vi "Real_Time_Main_Final.vi"() -> ()   [LabVIEW 2024]
uses:
  <instrlib>/niScope/Controls/niScope trigger source.ctl
  <vilib>/Platform/TimedLoop/XDataNode/timing_clust.ctl
  <vilib>/Platform/TimedLoop/XDataNode/nitl_modes.ctl
  <vilib>/Platform/TimedLoop/XDataNode/wakeup.ctl
  <instrlib>/niScope/Controls/niScope vertical coupling.ctl
  <instrlib>/niScope/Controls/niScope timestamp type.ctl
  <instrlib>/niScope/Configure/Trigger/niScope Configure Trigger Edge.vi
  <instrlib>/niScope/Acquire/Fetch/niScope Fetch WDT.vi
  <vilib>/platform/TimedLoop/XDataNode/XDataNode.xnode
  <vilib>/Platform/TimedLoop/XDataNode/XDNodeRunTimeDep.lvlib
panel:
  in  "stop 2":bool
  in  "Fetch:Fetch Relative To":i32(ring)=482 items=["Start"=482, "Trigger"=483, "Pretrigger"=477, "Now"=481, "Read Pointer"=388]
  in  "stop":bool
  out "error out":errorcluster
  out "Horizontal:Actual Sample Rate":dbl
  in  "channels":string="0"
  out "# of Points Fetched":i32
  out "# of Chunks Fetched":i32
  in  "trigger source":T1="0" caption="trigger source (Channel 0)"
  in  "Resource Name":refnum<k15>="Dev1" caption="Resource Name(s)"
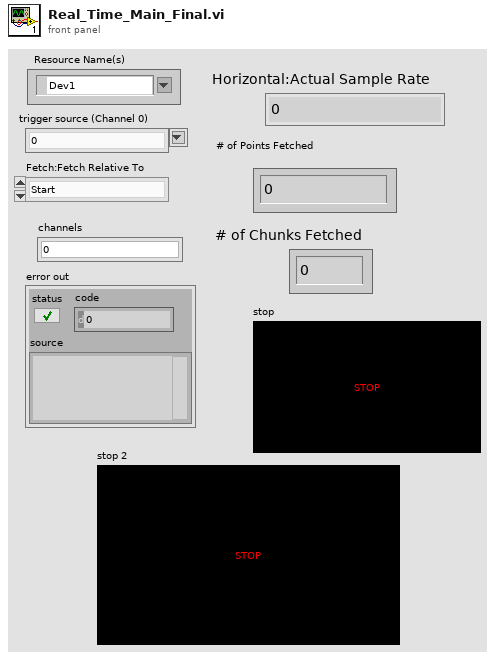
[diagram p1: front panel]
types:
  T1 = typedef "niScope trigger source.ctl" = string
  T2 = typedef "XDNodeRunTimeDep.lvlib/timing_clust.ctl" = cluster{"Expected End [f-1]":u64, "Actual End [f-1]":u64, "Finished Late? [f-1]":bool, "Expected End [i-1]":u64, "Actual End [i-1]":u64, "Finished Late? [i-1]":bool, "Expected Start [i]":u64, "Actual Start [i]":u64, "Expected Start [f]":u64, "Actual Start [f]":u64, "Source Name":string, "Structure Name":string, "Period":i64, "Deadline":i64, "Offset":i64, "Start":i64, "Priority":i32, "Timeout":i32, "Mode":T3, "Wakeup Reason":T4, "Error":errorcluster, "Source Type":string, "Secondary Source Type":string, "Global End Time":u64, "Global Start Time":u64, "Frame Duration":u64, "Iteration Duration":u64, "Assigned CPU":i32, "I/O Scan Engine Mode":u32}
  T3 = typedef "XDNodeRunTimeDep.lvlib/nitl_modes.ctl" = enum32{"No Change", "Process missed periods, maintain original phase", "Discard missed periods, maintain original phase", "Process missed periods, ignore original phase", "Discard missed periods, ignore original phase"}
  T4 = typedef "XDNodeRunTimeDep.lvlib/wakeup.ctl" = enum32{"Normal", "Aborted", "Asynchronous wakeup", "Timing source error", "Timed loop error", "Timeout"}
  T5 = typedef "niScope timestamp type.ctl" = i32
  T6 = typedef "niScope vertical coupling.ctl" = i32
  T7 = cluster{"actualSamples":i32, "absoluteInitialX":dbl, "relativeInitialX":dbl, "xIncrement":dbl, "offset":dbl, "gain":dbl, "reserved1":dbl, "reserved2":dbl}
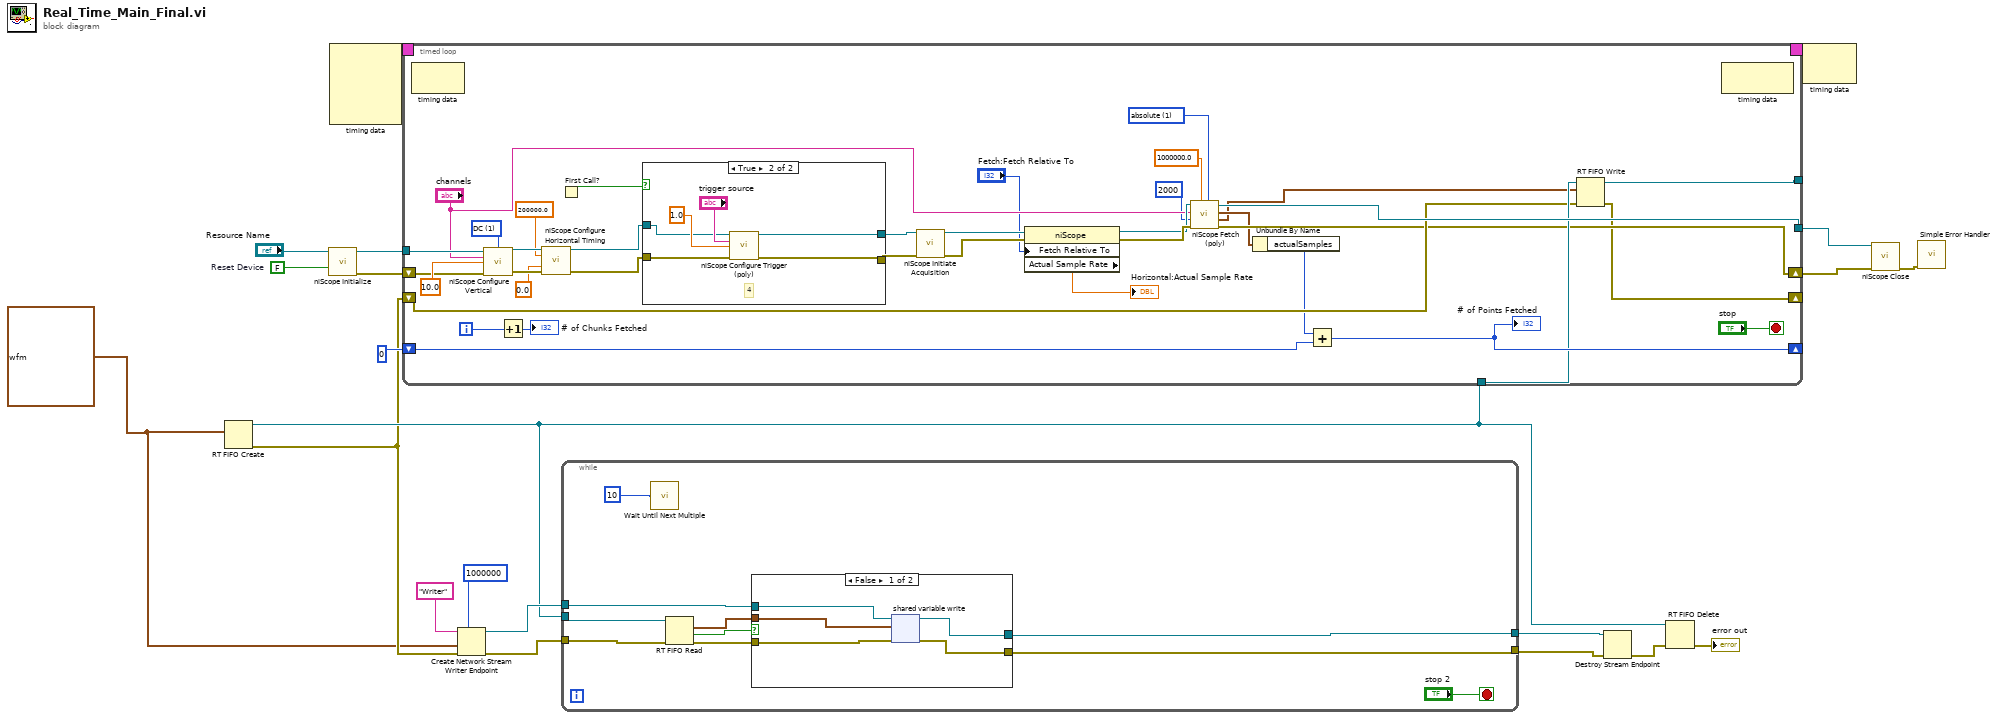
[diagram p0: block diagram]
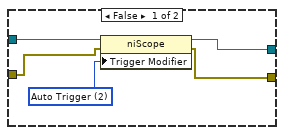
[diagram p3: hidden frame]
diagram:
  w1 = waveform(dbl) {"t0"=timestamp(0 s since 1904-01-01), "dt"=1.0, "Y"=[]}
  w21 = FALSE  # Reset Device
  n1 = RT FIFO Create(1:w1) -> (8:w6:refnum<k33>, 11:w3:errorcluster)  [unwired: 7 in, 1 out]
  n2 = call <instrlib>:"niScope Initialize.vi"("resource name"="Resource Name", "reset device"=w21) -> ("instrument handle"=w15:refnum<k15>, "error out"=w5:errorcluster)  [unwired: 12 in]
  n3 = node-c288() -> (w19:T2)  [unwired: 4 in]
  n4 = timed-loop {
    timing: w19 -> [_]
    timing-out: [_] -> w18
    tunnel: [w49] -> w17
    shift-right: [w47] -> _
    shift-left: 0 -> [w48]
    tunnel: w15 -> [w38]
    tunnel: w6 -> [w34]
    tunnel: [w33] -> _
    shift-right: [w26] -> _
    shift-left: w3 -> [w29]
    shift-right: [w27] -> w4
    shift-left: w5 -> [w28]
    i -> [w46]
    stop <- "stop" stop-if-true
    w23 = T5 1 items=["relative", "absolute"] ("timestamp Type")
    w42 = T6 1 items=["AC", "DC", "Ground"] ("vertical coupling")
    n5 = node-c288() -> ()  [unwired: 1 in, 1 out]
    n6 = call <instrlib>:"niScope Configure Vertical.vi"("instrument handle"=w38, "vertical coupling"=w42, "channels"="channels", "vertical range"=10.0, "error in"=w28) -> ("instrument handle out"=w45:refnum<k15>, "error out"=w39:errorcluster)  [unwired: 9 in]
    n7 = Increment(x=w46) -> (x+1=→"# of Chunks Fetched":i32)
    n8 = call <instrlib>:"niScope Configure Horizontal Timing.vi"("instrument handle"=w45, "min sample rate"=200000.0, "reference position"=0.0, "error in"=w39) -> ("instrument handle out"=w40:refnum<k15>, "error out"=w41:errorcluster)  [unwired: 10 in]
    n9 = First Call?() -> (First Call?: T/F=w57:bool)
    n10 = case shown="True" w57 {
      tunnel: [w62 w67] -> w58
      tunnel: [w63 w66] -> w51
      tunnel: w41 -> [w60 w65]
      tunnel: w40 -> [w59 w64]
      frame False {
        w61 = 2 items=["None"=1, "Auto Trigger"=2] ("Triggering:Trigger Modifier")
        n11 = property class="niScope"(reference=w59, error in=w60, "Trigger Modifier"=w61) -> (reference out=w63:refnum<k15>, error out=w62:errorcluster)
      }
      frame True {
        # "4"
        n12 = call-poly <instrlib>:"niScope Configure Trigger (poly).vi"("instrument handle"=w64, "trigger source"="trigger source", "trigger level"=1.0, "error in"=w65) -> ("instrument handle out"=w66:refnum<k15>, "error out"=w67:errorcluster)  [unwired: 10 in]
      }
    }
    n13 = call <instrlib>:"niScope Initiate Acquisition.vi"("instrument handle"=w51, "error in"=w58) -> ("instrument handle out"=w52:refnum<k15>, "error out"=w56:errorcluster)  [unwired: 12 in]
    n14 = property class="niScope"(reference=w52, error in=w56, "Fetch Relative To"="Fetch:Fetch Relative To") -> (reference out=w53:refnum<k15>, error out=w54:errorcluster, "Actual Sample Rate"=→"Horizontal:Actual Sample Rate":dbl)
    n15 = call-poly <instrlib>:"niScope Fetch (poly).vi"("timestamp Type"=w23, "timeout"=1000000.0, "error in"=w54, "numSamples"=2000, "channels"="channels", "instrument handle"=w53) -> ("error out"=w27:errorcluster, "wfm"=w22:waveform(dbl), "wfm info"=w25:T7, "instrument handle out"=w49:refnum<k15>)  [unwired: 2 in]
    n16 = Unbundle By Name(w25) -> ("actualSamples"=w24:i32)
    n17 = Add(x=w24, y=w48) -> (x+y=w47:i32)
    "# of Points Fetched" <- w47
    n18 = RT FIFO Write(0:w34, 1:w22, 3:w29) -> (8:w33:refnum<k33>, 11:w26:errorcluster)  [unwired: 2 in, 2 out]
    n19 = node-c288() -> ()  [unwired: 1 in, 1 out]
  }
  n20 = Create Network Stream Writer Endpoint(7:1000000 ("writer buffer size"), 8:w3, 9:w1, 11:"Writer" ("writer name")) -> (0:w12:errorcluster, 3:w11:refnum<k21>)  [unwired: 3 in]
  n21 = while {
    tunnel: w12 -> [w81]
    tunnel: w6 -> [w78]
    tunnel: w11 -> [w76]
    tunnel: [w73] -> w2
    tunnel: [w74] -> w7
    stop <- "stop 2" stop-if-true
    n22 = call "Wait Until Next Multiple"("Count(mSec)"=u32 10) -> ()  [unwired: 1 out]
    n23 = RT FIFO Read(0:w78, 3:w81) -> (9:w79:waveform(dbl), 10:w80:bool, 11:w77:errorcluster)  [unwired: 2 in, 2 out]
    n24 = case shown="False" w80 {
      tunnel: w79 -> [w82 _]
      tunnel: w77 -> [w83 w87]
      tunnel: w76 -> [w84 w88]
      tunnel: [w85 w87] -> w73
      tunnel: [w86 w88] -> w74
      frame False {
        n25 = shared-variable-write(w84, w83, w82) -> (w86:refnum<k21>, w85:errorcluster)  [unwired: 1 in, 1 out]
      }
      frame True {
      }
    }
  }
  n26 = Destroy Stream Endpoint(8:w2, 11:w7) -> (0:w10:errorcluster)
  n27 = RT FIFO Delete(0:w6, 3:w10) -> (11:→"error out":errorcluster)  [unwired: 1 in]
  n28 = node-c288(w18) -> ()  [unwired: 1 out]
  n29 = call <instrlib>:"niScope Close.vi"("instrument handle"=w17, "error in"=w4) -> ("error out"=w8:errorcluster)  [unwired: 13 in]
  n30 = call <vilib>:"Simple Error Handler.vi"("error in (no error)"=w8) -> ()  [unwired: 4 in, 5 out]
